vi "Get Instrument ID.vi"(8 "error in":errorcluster, 11 "VISA resource name in":refnum<visa-resource-name>) -> (0 "error out":errorcluster, 2 "instrument ID":string, 3 "VISA resource name out":refnum<visa-resource-name>)   [LabVIEW 2025, in "Chroma 19572.lvlib"]
uses:
  <instrlib>/Chroma 19572/Chroma 19572.lvlib
  <vilib>/Utility/error.llb/Trim Whitespace One-Sided.vi
panel:
  # "The CHROMA 19572 does not return the Serial Number with IDN?.\nThis VI provides the identification string including the Serial Number."
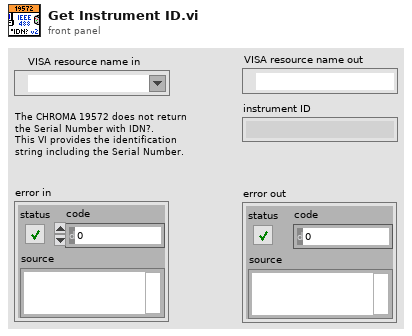
[diagram p1: front panel]
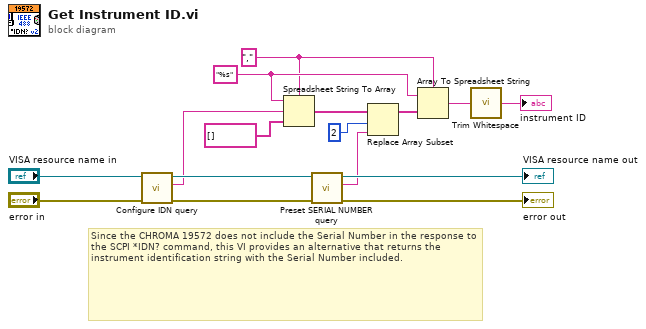
[diagram p0: block diagram]
diagram:
  w10 = "," ("delimiter (Tab)")
  w11 = "%s" ("format string")
  # "Since the CHROMA 19572 does not include the Serial Number in the response to the SCPI *IDN? command, this VI provides an alternative that returns the instrument identification string with the Serial Number included."
  n1 = call <instrlib>:"Configure IDN query.vi"("error in (no error)"="error in", "VISA resource name"="VISA resource name in") -> ("error out"=w4:errorcluster, "Result"=w2:string, "VISA resource name out"=w3:refnum<visa-resource-name>)  [unwired: 7 in]
  n2 = Spreadsheet String To Array(delimiter (Tab)=w10, format string=w11, spreadsheet string=w2, array type (2D Dbl)=string[] []) -> (array=w7:string[])
  n3 = call <instrlib>:"Preset SERIAL NUMBER query.vi"("error in (no error)"=w4, "VISA Refnum in"=w3) -> ("error out"=→"error out":errorcluster, "SERIAL number"=w5:string, "VISA Refnum out"=→"VISA resource name out":refnum<visa-resource-name>)  [unwired: 7 in]
  n4 = Replace Array Subset(array=w7, new element=w5, index=2) -> (w9:string[])
  n5 = Array To Spreadsheet String(delimiter (Tab)=w10, array=w9, 3:w11) -> (spreadsheet string=w1:string)
  n6 = call <vilib>:"Trim Whitespace.vi"("string"=w1) -> ("trimmed string"=→"instrument ID":string)  [unwired: 1 in]
